vi "Scan Setup.vi"(8 "error in (no error)":errorcluster, 11 "Translation Stage Fine in":refnum<class "Translation Stage Fine.lvclass">) -> (0 "error out":errorcluster, 3 "Translation Stage Fine out":refnum<class "Translation Stage Fine.lvclass">)   [LabVIEW 2012, in "Translation Stage Fine.lvclass"]
doc: "Configure the Instrument based on the class member fields. This step comes after the user has closed the \"Scan Setup\" window and before the actual scan -- so instruments are configured with the user's specified settings."
uses:
  Translation Stage Fine.lvclass
  Scanner/Scanner.lvclass
  Translation Stage Fine.lvclass/Translation Stage Fine.ctl
  Global/GPIB Numbers.vi
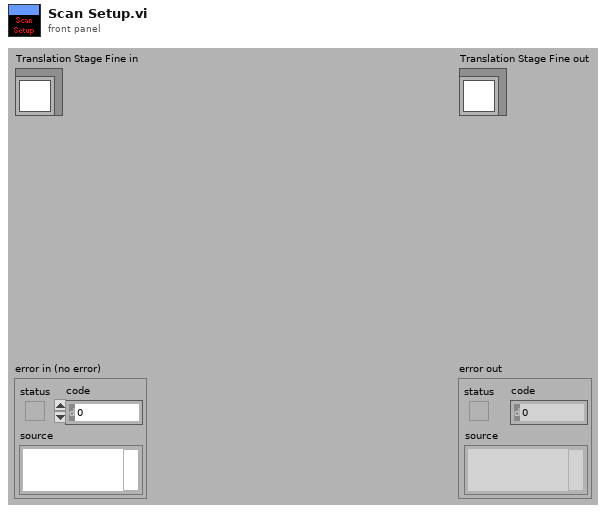
[diagram p1: front panel]
types:
  T1 = typedef "GPIB Type Def.ctl" = cluster{"Name":string, "bus":dbl, "GPIB":dbl, "GPIB as string":string, "byte":i32, "VISA Resource Name":refnum<visa-resource-name>}
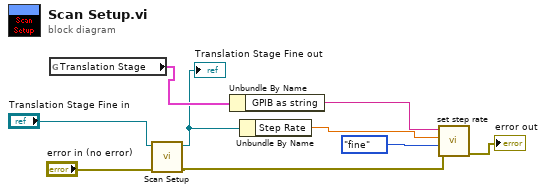
[diagram p0: block diagram]
diagram:
  n1 = global read "GPIB Numbers.vi" "Translation Stage"() -> (w4:T1)
  n2 = call-parent "Scan Setup.vi"("error in (no error)"="error in (no error)", "Scanner in"="Translation Stage Fine in") -> ("error out"=w2:errorcluster, "Scanner out"=w3:refnum<class "Translation Stage Fine.lvclass">)  [unwired: 8 in]
  "Translation Stage Fine out" <- w3
  n3 = Unbundle By Name(w4) -> ("GPIB as string"=w5:string)
  n4 = Unbundle By Name(w3) -> ("Step Rate"=w6:dbl)
  n5 = call "set step rate.vi"("error in"=w2, "axis (def: fine)"=enum16{"fine", "coarse"}."fine", "step rate"=w6, "GPIB # (in): def. 6"=w5) -> ("error out"=→"error out":errorcluster)  [unwired: 7 out]
